vi "Material-Overall-P_F.vi"(8 "error in":errorcluster, 11 "Material-RunTest in":refnum<class "Material-RunTest.lvclass">) -> (0 "error out":errorcluster, 2 "Sheet Overall Passed?":bool, 3 "Material-RunTest in 2":refnum<class "Material-RunTest.lvclass">)   [LabVIEW 2013, in "Material-RunTest.lvclass"]
uses:
  Material-RunTest.lvclass
  Material-RunTest.lvclass/Material-RunTest.ctl
  <userlib>/_MGI/1D Array/MGI Average/MGI Average (DBL[]).vi
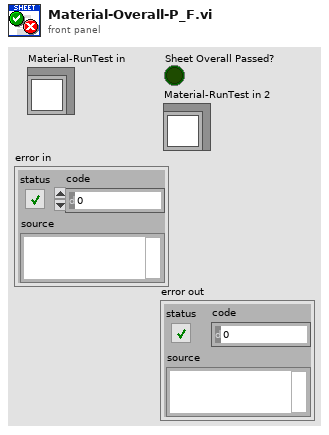
[diagram p1: front panel]
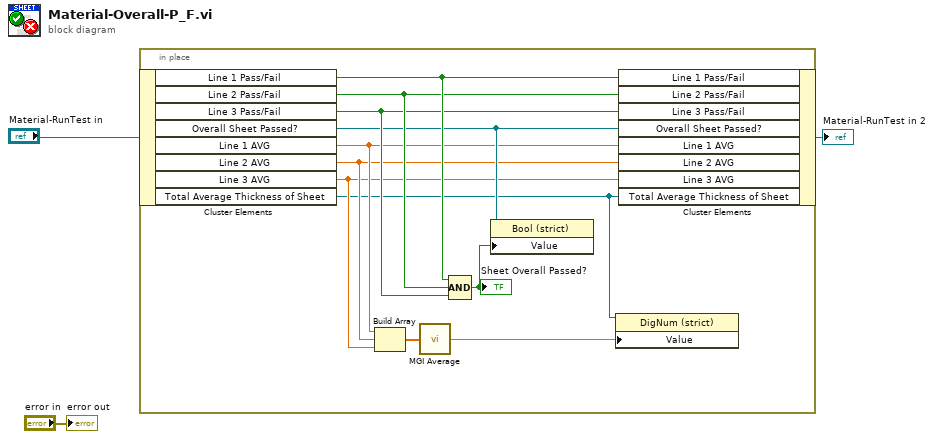
[diagram p0: block diagram]
diagram:
  n1 = in-place {
    n2 = in-place-cluster #1("Material-RunTest in") -> ("Line 1 Pass/Fail"=w14:bool, "Line 2 Pass/Fail"=w13:bool, "Line 3 Pass/Fail"=w12:bool, "Overall Sheet Passed?"=w10:refnum<vi>, "Line 1 AVG"=w9:dbl, "Line 2 AVG"=w8:dbl, "Line 3 AVG"=w7:dbl, "Total Average Thickness of Sheet"=w4:refnum<vi>)
    n3 = Build Array(w9, w8, w7) -> (w6:dbl[])
    n4 = call-poly <userlib>:"MGI Average.vi"("Double[]"=w6) -> ("Average"=w5:dbl)  [unwired: 1 in]
    n5 = Compound Arithmetic op=AND(w14, w13, w12) -> (w11:bool)
    "Sheet Overall Passed?" <- w11
    n6 = property class="Bool (strict)"(reference=w10, "Value"=w11) -> ()  [unwired: 1 in, 2 out]
    n7 = property class="DigNum (strict)"(reference=w4, "Value"=w5) -> ()  [unwired: 1 in, 2 out]
    n8 = in-place-cluster #1("Line 1 Pass/Fail"=w14, "Line 2 Pass/Fail"=w13, "Line 3 Pass/Fail"=w12, "Overall Sheet Passed?"=w10, "Line 1 AVG"=w9, "Line 2 AVG"=w8, "Line 3 AVG"=w7, "Total Average Thickness of Sheet"=w4) -> (→"Material-RunTest in 2":refnum<class "Material-RunTest.lvclass">)
  }
  "error out" <- "error in"
